vi "Initialize Channel Manager Array.vi"(8 "error in (no error)":errorcluster, 11 "SPARC4_AC in":refnum<class "S4ACS_GUI.lvclass">) -> (0 "error out":errorcluster, 3 "SPARC4_AC out":refnum<class "S4ACS_GUI.lvclass">)   [LabVIEW 2012, in "S4ACS_GUI.lvclass"]
uses:
  S4ACS_GUI.lvclass
  SPARC4 - 12-11-2020/SPARC4 GUI test/SPARC4/SPARC4_GUI/Channel Manager/Channel Manager.lvclass
panel:
  in  "Channel Manager.lvclass":refnum<class "Channel Manager.lvclass">=refnum
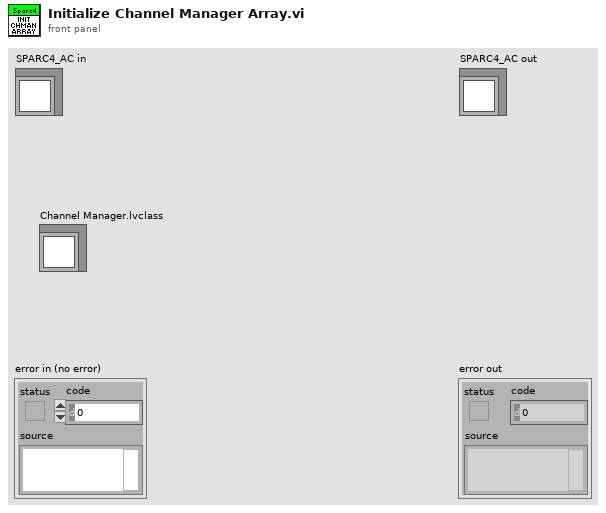
[diagram p1: front panel]
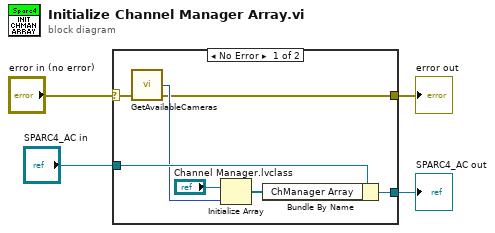
[diagram p0: block diagram]
diagram:
  n1 = case shown="No Error" "error in (no error)" {
    selector: "error in (no error)" -> [w11 w13]
    tunnel: [w5 w13] -> w3
    tunnel: [w9 w12] -> w1
    tunnel: "SPARC4_AC in" -> [w10 w12]
    frame No Error {
      n2 = call "GetAvailableCameras.vi"("error in (no error)"=w11) -> ("error out"=w5:errorcluster, "totalCameras"=w7:i32)  [unwired: 2 in, 1 out]
      n3 = Initialize Array("Channel Manager.lvclass", w7) -> (w6:refnum<class "Channel Manager.lvclass">[])
      n4 = Bundle By Name(cluster=w10, "ChManager Array"=w6) -> (w9:refnum<class "S4ACS_GUI.lvclass">)
    }
    frame Error {
    }
  }
  "error out" <- w3
  "SPARC4_AC out" <- w1
